vi "main.vi"() -> ()   [LabVIEW 2015]
uses:
  Solution/Controls/Buttons.ctl
  Solution/Controls/Menu.ctl
  Controls/Orders.ctl
  Controls/state.ctl
  Controls/Actiob.ctl
  Controls/useraction.ctl
  Controls/message.ctl
  Controls/Filestate.ctl
  Controls/Users data.ctl
  Controls/user.ctl
panel:
  in  "Right Buttons":T1
  out "Right Menu":T2
  out "Left Menu":T2
  out "ATM Messages":string
  in  "User Input":string
  in  "Enter":bool
  in  "Left Buttons":T1
  in  "Card Simulator":bool
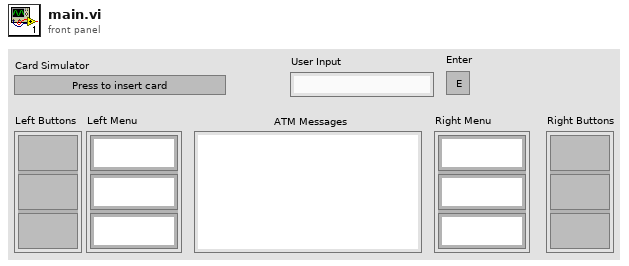
[diagram p1: front panel]
types:
  T1 = typedef "Buttons.ctl" = cluster{"Button 0":bool, "Button 1":bool, "Button 2":bool}
  T2 = typedef "Menu.ctl" = cluster{"Menu 0":string, "Menu 1":string, "Menu 2":string}
  T3 = typedef "Orders.ctl" = cluster{"state":T4, "Action":T5, "Data":string}
  T4 = typedef "state.ctl" = enum16{"Error", "Insert Card", "Initialize", "Enter", "Fast Cash", "Withdraw", "Deposit", "R&T", "Balance"}
  T5 = typedef "Actiob.ctl" = enum16{"Validate", "Deposit", "Withdraw"}
  T6 = enum8{"Enabled", "Disabled", "Disabled and Grayed Out"}
  T7 = typedef "useraction.ctl" = enum16{"Balance", "Withdraw", "Deposit"}
  T8 = typedef "message.ctl" = enum16{"Deposit Complete", "Welcome", "Menu", "Verification Failed", "Session Terminate", "Deposit", "Withdrawal", "Withdrawal Complete", "Withdrawal Failed", "Balance Inq"}
  T9 = typedef "Filestate.ctl" = enum16{"Read", "Write"}
  T10 = typedef "Users data.ctl" = cluster{"Users ":T11[], "User ind":i32}
  T11 = typedef "user.ctl" = cluster{"Full Name":string, "Code":string, "Money":string}
  T12 = cluster{"RFS String":string, "RFS String 2":string, "RFS String 3":string}
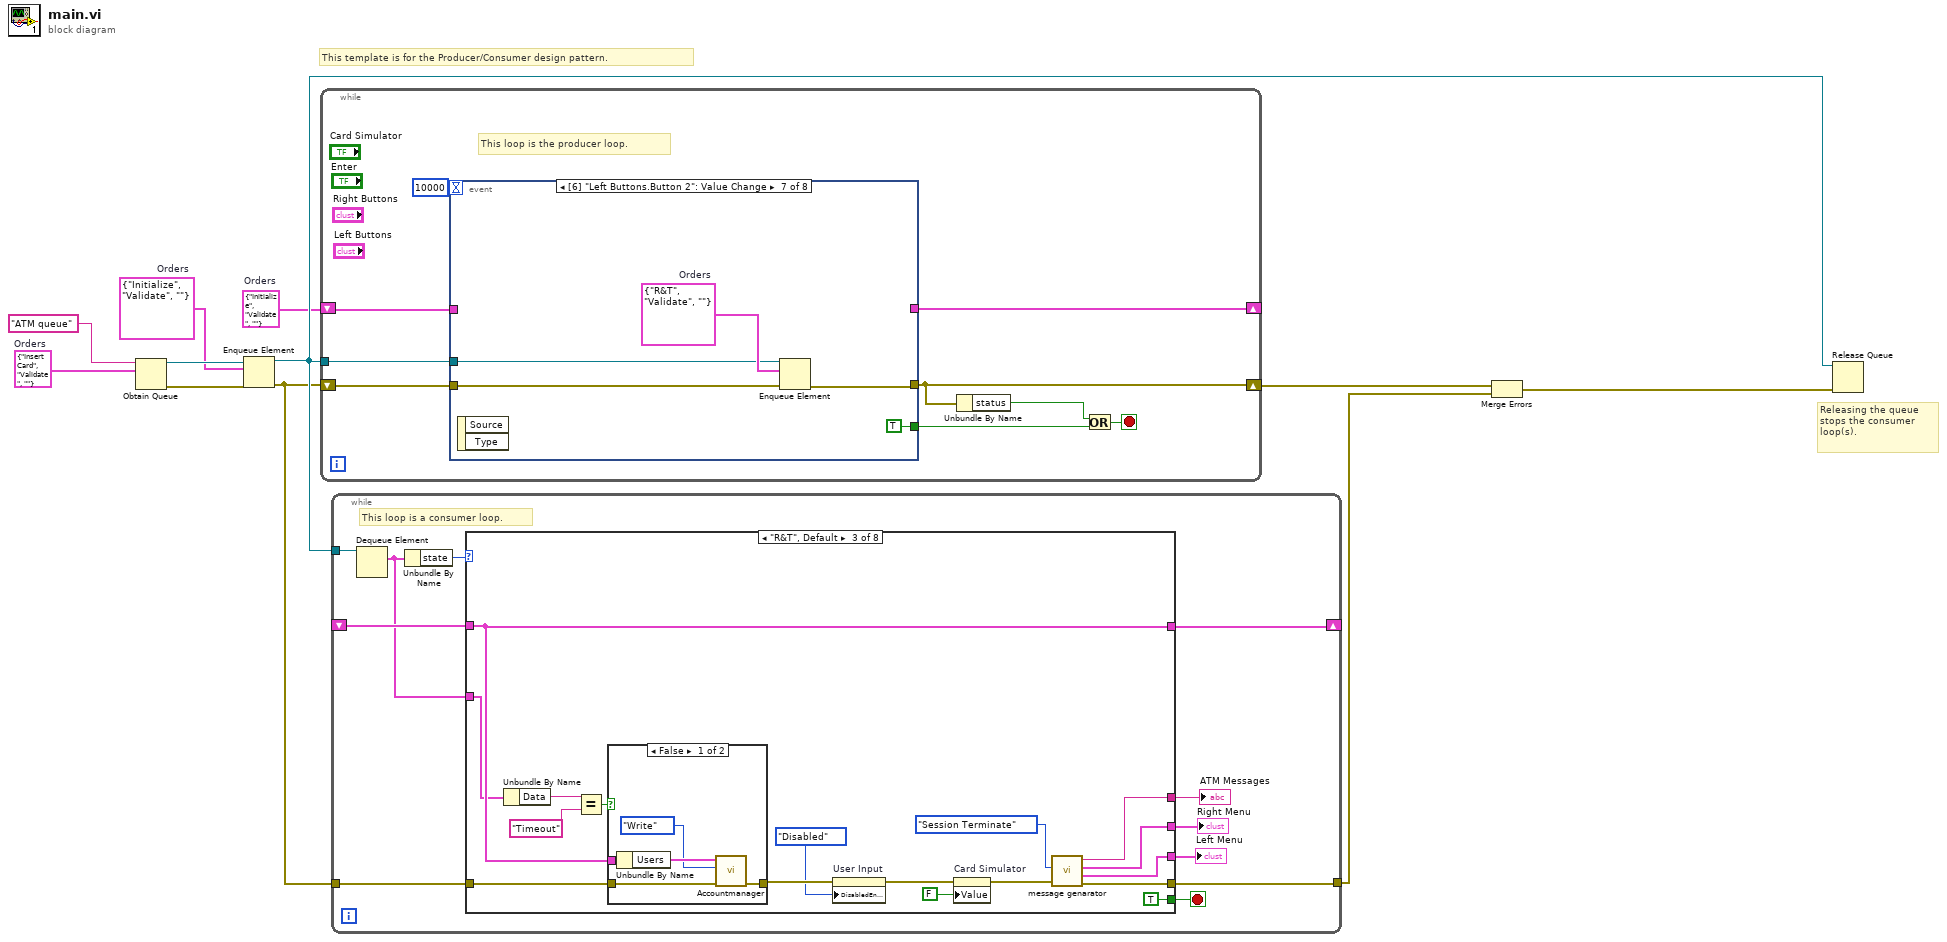
[diagram p0: block diagram]
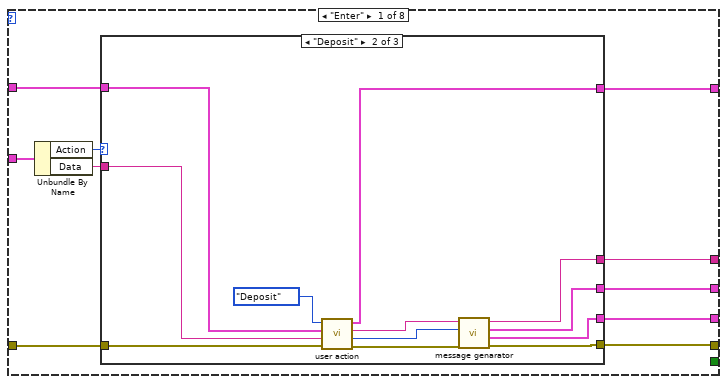
[diagram p2: hidden frame]
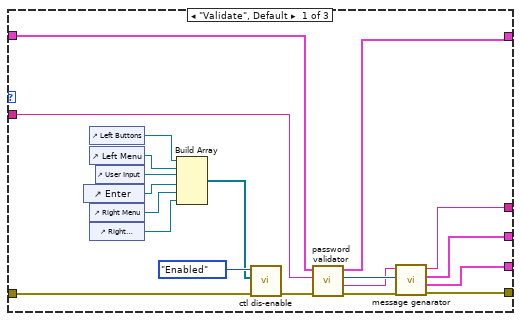
[diagram p3: hidden frame]
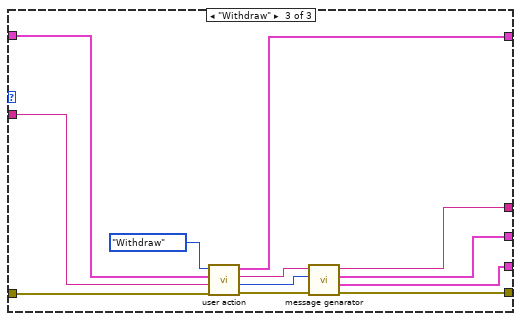
[diagram p4: hidden frame]
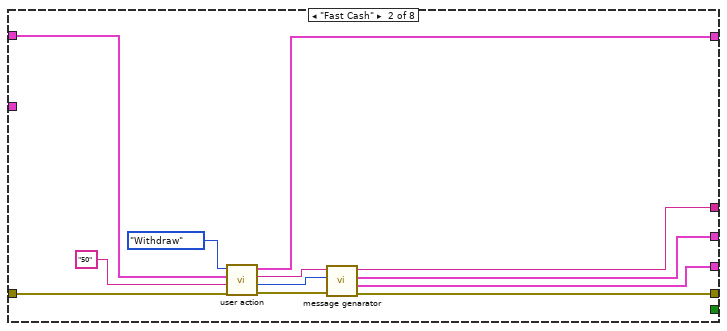
[diagram p5: hidden frame]
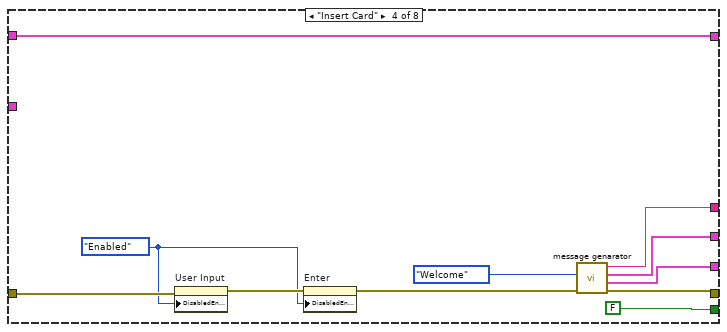
[diagram p7: hidden frame]
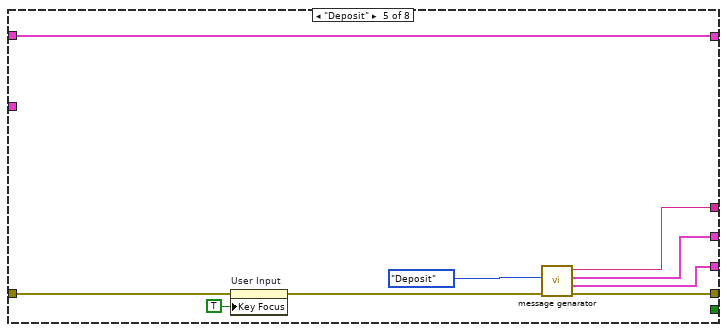
[diagram p8: hidden frame]
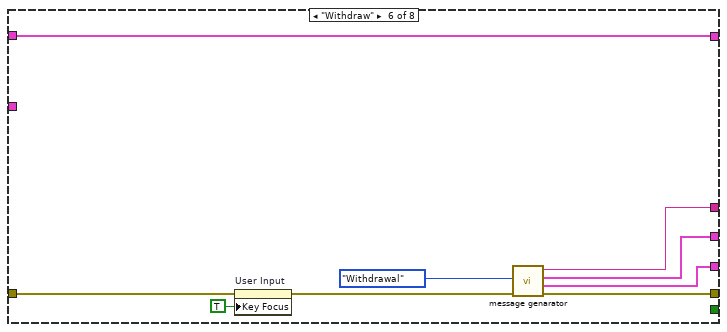
[diagram p9: hidden frame]
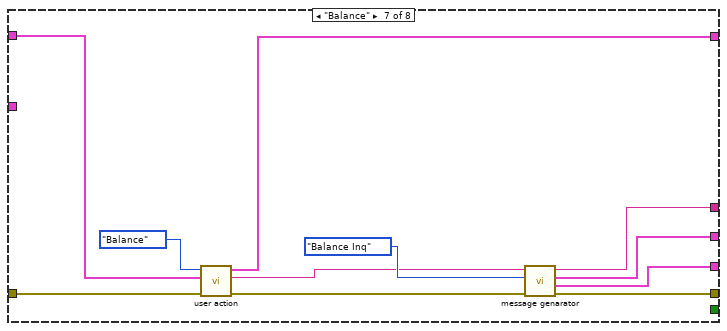
[diagram p10: hidden frame]
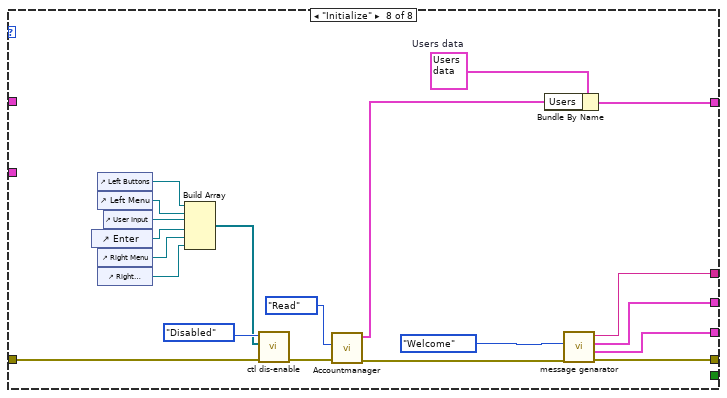
[diagram p11: hidden frame]
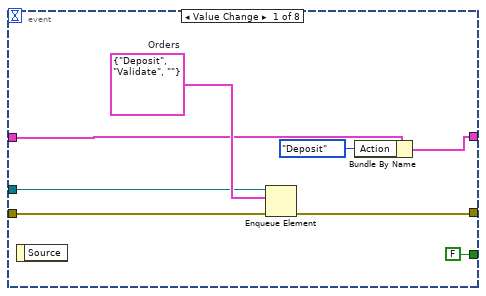
[diagram p12: hidden frame]
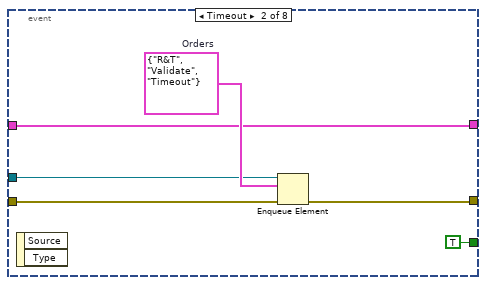
[diagram p13: hidden frame]
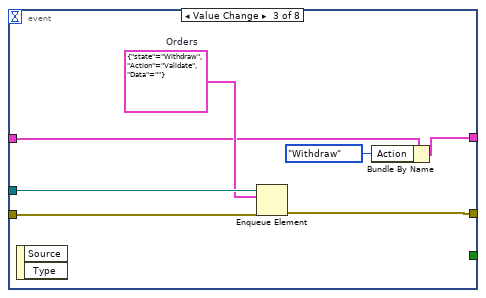
[diagram p14: hidden frame]
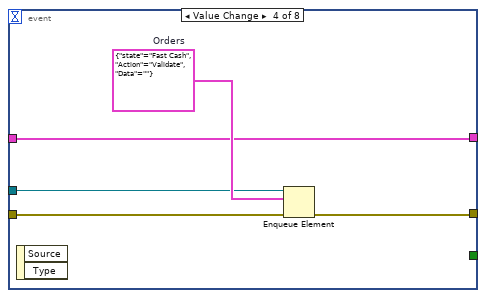
[diagram p15: hidden frame]
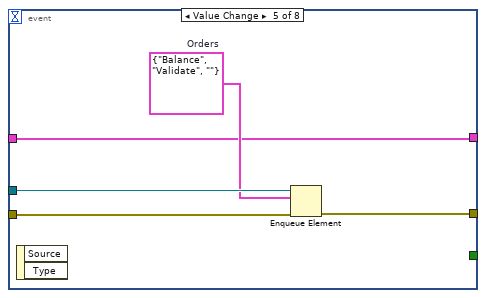
[diagram p16: hidden frame]
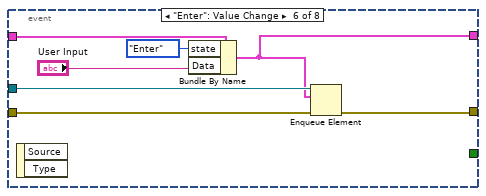
[diagram p17: hidden frame]
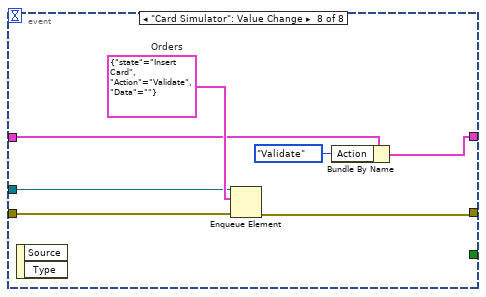
[diagram p18: hidden frame]
diagram:
  w4 = T3 {"state"=enum."Initialize", "Action"=enum."Validate", "Data"=""}  # Orders
  w6 = T3 {"state"=enum."Initialize", "Action"=enum."Validate", "Data"=""}  # Orders
  w11 = T3 {"state"=enum."Insert Card", "Action"=enum."Validate", "Data"=""}  # Orders
  # "Releasing the queue stops the consumer loop(s)."
  # "This template is for the Producer/Consumer design pattern."
  n1 = Obtain Queue(name (unnamed)="ATM queue", element data type=w11) -> (queue out=w8:refnum<queue>, error out=w9:errorcluster)  [unwired: 3 in, 1 out]
  n2 = Enqueue Element(queue=w8, element=w6, error in (no error)=w9) -> (queue out=w7:refnum<queue>, error out=w5:errorcluster)  [unwired: 1 in, 1 out]
  n3 = while {
    shift-right: [w16] -> w3
    shift-left: w5 -> [w19]
    tunnel: w7 -> [w20]
    shift-right: [w13] -> _
    shift-left: w4 -> [w14]
    stop <- w17 stop-if-true
    # "This loop is the producer loop."
    n4 = event shown="[6] \"Left Buttons.Button 2\": Value Change" {
      selector: _ -> [_ _ _ _ _ _ _ _]
      dyn-events: _ -> [_ _ _ _ _ _ _ _]
      timeout: 10000 -> [_ _ _ _ _ _ _ _]
      tunnel: w20 -> [w24 w31 w39 w43 w49 w56 w60 w67]
      tunnel: w19 -> [w27 w34 w41 w46 w51 w55 w63 w70]
      tunnel: [w26 w33 w40 w45 w50 w54 w62 w68] -> w16
      tunnel: [FALSE ("stop") TRUE ("stop") _ _ _ _ TRUE ("stop") _] -> w18
      tunnel: w14 -> [w23 w30 w37 w42 w47 w58 _ w66]
      tunnel: [w21 w30 w36 w42 w47 w53 _ w64] -> w13
      event Value Change {
        w25 = T3 {"state"=enum."Deposit", "Action"=enum."Validate", "Data"=""}  # Orders
        n5 = event-data() -> ()  [unwired: 1 in, 1 out]
        n6 = Enqueue Element(queue=w24, element=w25, error in (no error)=w27) -> (error out=w26:errorcluster)  [unwired: 1 in, 2 out]
        n7 = Bundle By Name(cluster=w23, "Action"=Actiob."Deposit") -> (w21:T3)
      }
      event Timeout {
        w32 = T3 {"state"=enum."R&T", "Action"=enum."Validate", "Data"="Timeout"}  # Orders
        n8 = event-data() -> ()  [unwired: 1 in, 2 out]
        n9 = Enqueue Element(queue=w31, element=w32, error in (no error)=w34) -> (error out=w33:errorcluster)  [unwired: 1 in, 2 out]
      }
      event Value Change {
        w38 = T3 {"state"=enum."Withdraw", "Action"=enum."Validate", "Data"=""}  # Orders
        n10 = event-data() -> ()  [unwired: 1 in, 2 out]
        n11 = Enqueue Element(queue=w39, element=w38, error in (no error)=w41) -> (error out=w40:errorcluster)  [unwired: 1 in, 2 out]
        n12 = Bundle By Name(cluster=w37, "Action"=Actiob."Withdraw") -> (w36:T3)
      }
      event Value Change {
        w44 = T3 {"state"=enum."Fast Cash", "Action"=enum."Validate", "Data"=""}  # Orders
        n13 = event-data() -> ()  [unwired: 1 in, 2 out]
        n14 = Enqueue Element(queue=w43, element=w44, error in (no error)=w46) -> (error out=w45:errorcluster)  [unwired: 1 in, 2 out]
      }
      event Value Change {
        w48 = T3 {"state"=enum."Balance", "Action"=enum."Validate", "Data"=""}  # Orders
        n15 = event-data() -> ()  [unwired: 1 in, 2 out]
        n16 = Enqueue Element(queue=w49, element=w48, error in (no error)=w51) -> (error out=w50:errorcluster)  [unwired: 1 in, 2 out]
      }
      event "Enter": Value Change {
        n17 = event-data() -> ()  [unwired: 1 in, 2 out]
        n18 = Bundle By Name(cluster=w58, "state"=state."Enter", "Data"="User Input") -> (w53:T3)
        n19 = Enqueue Element(queue=w56, element=w53, error in (no error)=w55) -> (error out=w54:errorcluster)  [unwired: 1 in, 2 out]
      }
      event Value Change {
        w61 = T3 {"state"=enum."R&T", "Action"=enum."Validate", "Data"=""}  # Orders
        n20 = event-data() -> ()  [unwired: 1 in, 2 out]
        n21 = Enqueue Element(queue=w60, element=w61, error in (no error)=w63) -> (error out=w62:errorcluster)  [unwired: 1 in, 2 out]
      }
      event "Card Simulator": Value Change {
        w69 = T3 {"state"=enum."Insert Card", "Action"=enum."Validate", "Data"=""}  # Orders
        n22 = event-data() -> ()  [unwired: 1 in, 2 out]
        n23 = Enqueue Element(queue=w67, element=w69, error in (no error)=w70) -> (error out=w68:errorcluster)  [unwired: 1 in, 2 out]
        n24 = Bundle By Name(cluster=w66, "Action"=Actiob."Validate") -> (w64:T3)
      }
    }
    n25 = Unbundle By Name(w16) -> ("status"=w15:bool)
    n26 = Or(x=w15, y=w18) -> (x .or. y?=w17:bool)
  }
  n27 = while {
    tunnel: w7 -> [w81]
    tunnel: w5 -> [w78]
    tunnel: [w77] -> w2
    shift-right: [w73] -> _
    shift-left: _ -> [w72]
    stop <- w80 stop-if-true
    # "This loop is a consumer loop."
    n28 = Dequeue Element(queue=w81) -> (element=w71:T3)  [unwired: 2 in, 3 out]
    n29 = Unbundle By Name(w71) -> ("state"=w79:T4)
    n30 = case shown="\"R&T\", Default" w79 {
      tunnel: [_ _ TRUE FALSE _ _ _ _] -> w80
      tunnel: w78 -> [w88 w145 w164 w180 w190 w198 w210 w222]
      tunnel: [w85 w140 w163 w176 w186 w195 w208 w220] -> w77
      tunnel: [w84 w139 w162 w175 w185 w194 w200 w219] -> w76
      tunnel: [w83 w138 w161 w174 w184 w193 w201 w218] -> w75
      tunnel: [w82 w137 w160 w173 w183 w192 w202 w217] -> w74
      tunnel: [w86 w136 w159 w171 w182 w191 w205 w212] -> w73
      tunnel: w72 -> [w89 w142 w159 w171 w182 w191 w206 _]
      tunnel: w71 -> [w91 _ w158 _ _ _ _ _]
      frame "Enter" {
        n31 = Unbundle By Name(w91) -> ("Action"=w90:T5, "Data"=w87:string)
        n32 = case shown="\"Deposit\"" w90 {
          tunnel: w89 -> [w110 w118 w132]
          tunnel: w88 -> [w92 w123 w134]
          tunnel: w87 -> [w111 w117 w133]
          tunnel: [w109 w119 w128] -> w86
          tunnel: [w105 w115 w127] -> w85
          tunnel: [w104 w114 w126] -> w84
          tunnel: [w103 w113 w125] -> w83
          tunnel: [w102 w112 w124] -> w82
          frame "Validate", Default {
            n33 = control-ref of="Enter"() -> (w97:refnum<vi>)
            n34 = control-ref of="Left Buttons"() -> (w94:refnum<vi>)
            n35 = control-ref of="Left Menu"() -> (w95:refnum<vi>)
            n36 = control-ref of="Right Menu"() -> (w98:refnum<vi>)
            n37 = control-ref of="Right Buttons"() -> (w99:refnum<vi>)
            n38 = control-ref of="User Input"() -> (w96:refnum<vi>)
            n39 = Build Array(w94, w95, w96, w97, w98, w99) -> (w100:refnum<vi>[])
            n40 = call "ctl dis-enable.vi"("error in"=w92, "Array"=w100, "Disabled"=T6."Enabled") -> ("error out"=w93:errorcluster)  [unwired: 8 in]
            n41 = call "password validator.vi"("error in"=w93, "User Input"=w111, "Users data"=w110) -> ("error out"=w108:errorcluster, "Full Name"=w106:string, "Message out"=w107:T8, "Users data out"=w109:T10)  [unwired: 5 in]
            n42 = call "message genarator.vi"("error in"=w108, "Message in"=w107, "Input data"=w106) -> ("error out"=w105:errorcluster, "Left Menu"=w104:T12, "Right Menu"=w103:T12, "Message out"=w102:string)  [unwired: 5 in]
          }
          frame "Deposit" {
            n43 = call "user action.vi"("error in"=w123, "Cash"=w117, "Users data"=w118, "user action"=useraction."Deposit") -> ("error out"=w122:errorcluster, "Messageout"=w121:T8, "Output"=w120:string, "Users data out"=w119:T10)  [unwired: 4 in]
            n44 = call "message genarator.vi"("error in"=w122, "Message in"=w121, "Input data"=w120) -> ("error out"=w115:errorcluster, "Left Menu"=w114:T12, "Right Menu"=w113:T12, "Message out"=w112:string)  [unwired: 5 in]
          }
          frame "Withdraw" {
            n45 = call "user action.vi"("error in"=w134, "Cash"=w133, "Users data"=w132, "user action"=useraction."Withdraw") -> ("error out"=w131:errorcluster, "Messageout"=w130:T8, "Output"=w129:string, "Users data out"=w128:T10)  [unwired: 4 in]
            n46 = call "message genarator.vi"("error in"=w131, "Message in"=w130, "Input data"=w129) -> ("error out"=w127:errorcluster, "Left Menu"=w126:T12, "Right Menu"=w125:T12, "Message out"=w124:string)  [unwired: 5 in]
          }
        }
      }
      frame "Fast Cash" {
        n47 = call "user action.vi"("error in"=w145, "Cash"="50", "Users data"=w142, "user action"=useraction."Withdraw") -> ("error out"=w144:errorcluster, "Messageout"=w143:T8, "Output"=w146:string, "Users data out"=w136:T10)  [unwired: 4 in]
        n48 = call "message genarator.vi"("error in"=w144, "Message in"=w143, "Input data"=w146) -> ("error out"=w140:errorcluster, "Left Menu"=w139:T12, "Right Menu"=w138:T12, "Message out"=w137:string)  [unwired: 5 in]
      }
      frame "R&T", Default {
        n49 = Unbundle By Name(w158) -> ("Data"=w156:string)
        n50 = Equal?(x=w156, y="Timeout") -> (x = y?=w155:bool)
        n51 = case shown="False" w155 {
          tunnel: w164 -> [w169 w170]
          tunnel: [w168 w170] -> w150
          tunnel: w159 -> [w165 _]
          frame False {
            n52 = Unbundle By Name(w165) -> ("Users"=w167:T11[])
            n53 = call "Accountmanager.vi"("error in (no error)"=w169, "Filestate"=Filestate."Write", "Users in"=w167) -> ("error out"=w168:errorcluster)  [unwired: 7 in, 1 out]
          }
          frame True {
          }
        }
        n54 = property on="User Input" class="Str"(error in=w150, "DisabledEnum"=T6."Disabled" ("Disabled")) -> (error out=w149:errorcluster)  [unwired: 1 in, 1 out]
        n55 = property on="Card Simulator" class="Bool (strict)"(error in=w149, "Value"=FALSE ("Card Simulator")) -> (error out=w151:errorcluster)  [unwired: 1 in, 1 out]
        n56 = call "message genarator.vi"("error in"=w151, "Message in"=message."Session Terminate") -> ("error out"=w163:errorcluster, "Left Menu"=w162:T12, "Right Menu"=w161:T12, "Message out"=w160:string)  [unwired: 6 in]
      }
      frame "Insert Card" {
        w172 = T6."Enabled" ("Disabled")
        n57 = property on="User Input" class="Str"(error in=w180, "DisabledEnum"=w172) -> (error out=w179:errorcluster)  [unwired: 1 in, 1 out]
        n58 = property on="Enter" class="Bool"(error in=w179, "DisabledEnum"=w172) -> (error out=w178:errorcluster)  [unwired: 1 in, 1 out]
        n59 = call "message genarator.vi"("error in"=w178, "Message in"=message."Welcome") -> ("error out"=w176:errorcluster, "Left Menu"=w175:T12, "Right Menu"=w174:T12, "Message out"=w173:string)  [unwired: 6 in]
      }
      frame "Deposit" {
        n60 = property on="User Input" class="Str"(error in=w190, "Key Focus"=TRUE) -> (error out=w187:errorcluster)  [unwired: 1 in, 1 out]
        n61 = call "message genarator.vi"("error in"=w187, "Message in"=message."Deposit") -> ("error out"=w186:errorcluster, "Left Menu"=w185:T12, "Right Menu"=w184:T12, "Message out"=w183:string)  [unwired: 6 in]
      }
      frame "Withdraw" {
        n62 = property on="User Input" class="Str"(error in=w198, "Key Focus"=TRUE) -> (error out=w197:errorcluster)  [unwired: 1 in, 1 out]
        n63 = call "message genarator.vi"("error in"=w197, "Message in"=message."Withdrawal") -> ("error out"=w195:errorcluster, "Left Menu"=w194:T12, "Right Menu"=w193:T12, "Message out"=w192:string)  [unwired: 6 in]
      }
      frame "Balance" {
        n64 = call "user action.vi"("error in"=w210, "Users data"=w206, "user action"=useraction."Balance") -> ("error out"=w209:errorcluster, "Output"=w203:string, "Users data out"=w205:T10)  [unwired: 5 in, 1 out]
        n65 = call "message genarator.vi"("error in"=w209, "Message in"=message."Balance Inq", "Input data"=w203) -> ("error out"=w208:errorcluster, "Left Menu"=w200:T12, "Right Menu"=w201:T12, "Message out"=w202:string)  [unwired: 5 in]
      }
      frame "Initialize" {
        w214 = T10 {"Users "=[{"Full Name"="John  Doe", "Code"="12345", "Money"="550"}, {"Full Name"="Jennifer  Rodriguez", "Code"="23456", "Money"="1000"}, {"Full Name"="Bryan  Smith", "Code"="34567", "Money"="750"}, {"Full Name"="Julie  Ramirez", "Code"="45678", "Money"="900"}], "User ind"=0}  # Users data
        n66 = control-ref of="Enter"() -> (w226:refnum<vi>)
        n67 = control-ref of="Left Buttons"() -> (w223:refnum<vi>)
        n68 = control-ref of="Left Menu"() -> (w224:refnum<vi>)
        n69 = control-ref of="Right Menu"() -> (w227:refnum<vi>)
        n70 = control-ref of="Right Buttons"() -> (w228:refnum<vi>)
        n71 = control-ref of="User Input"() -> (w225:refnum<vi>)
        n72 = Build Array(w223, w224, w225, w226, w227, w228) -> (w229:refnum<vi>[])
        n73 = call "ctl dis-enable.vi"("error in"=w222, "Array"=w229, "Disabled"=T6."Disabled") -> ("error out"=w216:errorcluster)  [unwired: 8 in]
        n74 = call "Accountmanager.vi"("error in (no error)"=w216, "Filestate"=Filestate."Read") -> ("error out"=w215:errorcluster, "Users out"=w213:T11[])  [unwired: 8 in]
        n75 = Bundle By Name(cluster=w214, "Users"=w213) -> (w212:T10)
        n76 = call "message genarator.vi"("error in"=w215, "Message in"=message."Welcome") -> ("error out"=w220:errorcluster, "Left Menu"=w219:T12, "Right Menu"=w218:T12, "Message out"=w217:string)  [unwired: 6 in]
      }
    }
    "ATM Messages" <- w74
    "Right Menu" <- w75
    "Left Menu" <- w76
  }
  n77 = Merge Errors(w3, w2) -> (w1:errorcluster)
  n78 = Release Queue(queue=w7, error in (no error)=w1) -> ()  [unwired: 1 in, 3 out]
